vi "Fibonacci LFSRs -pseudo random.vi"() -> (3 "rand number":u16)   [LabVIEW 2021]
doc: "genarate pasodo random number.\nhttps://en.wikipedia.org/wiki/Linear-feedback_shift_register"
panel:
  # "tested, its has a flat histogram!"
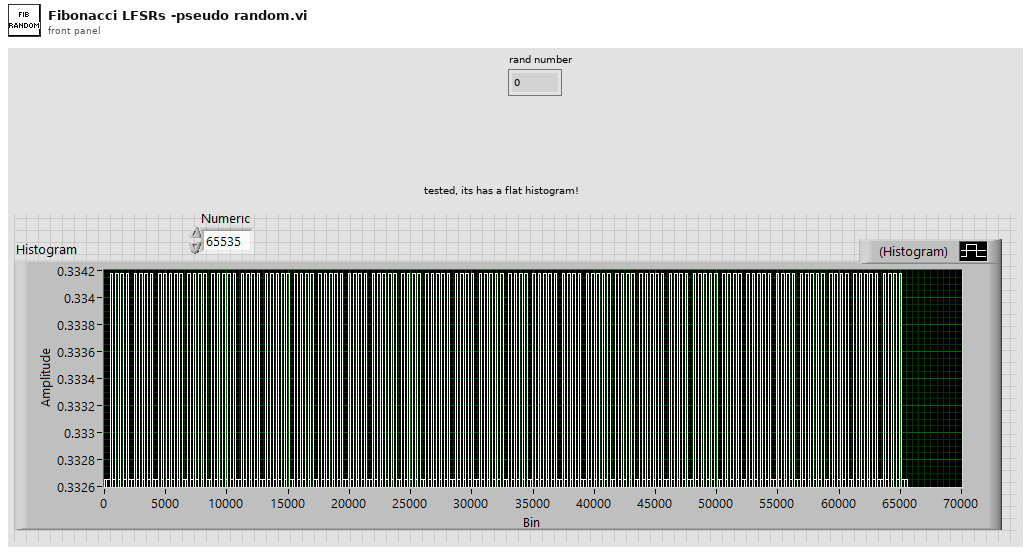
[diagram p1: front panel]
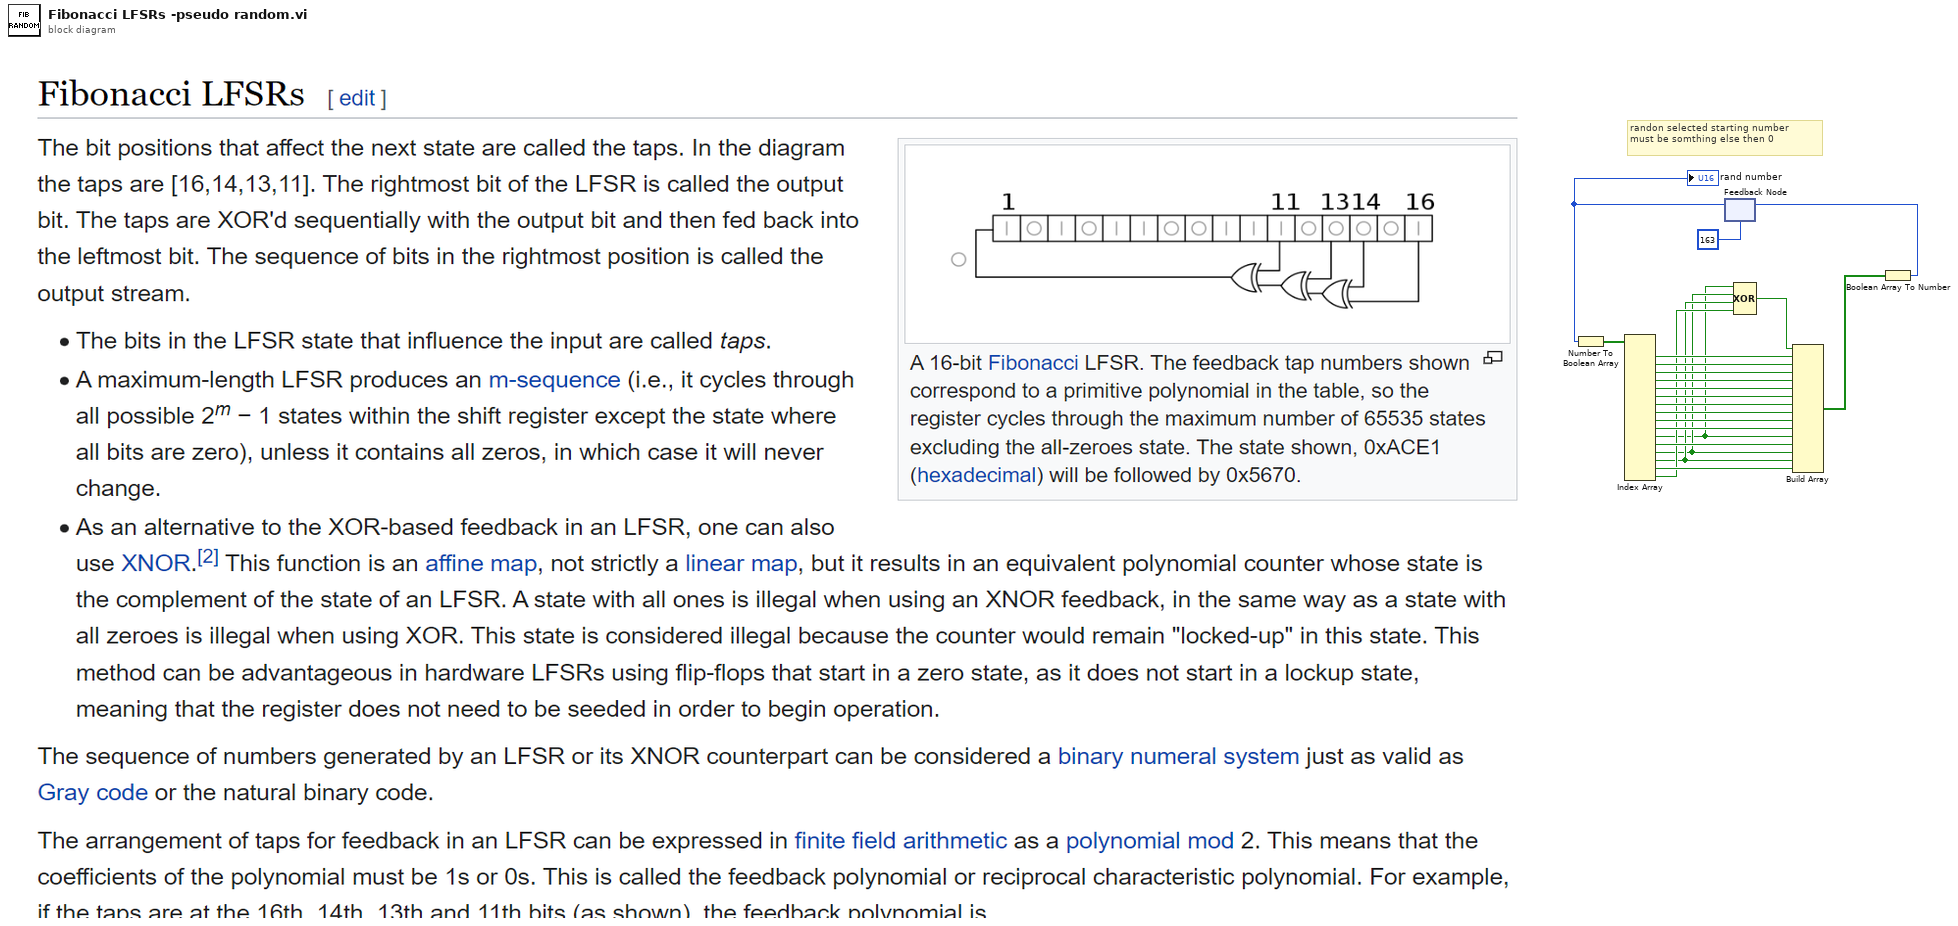
[diagram p0: block diagram]
diagram:
  # "randon selected starting number\nmust be somthing else then 0"
  n1 = feedback #1(u16 163) -> (w2:u16)
  "rand number" <- w2
  n2 = Number To Boolean Array(number=w2) -> (Boolean array=w22:bool[])
  n3 = Index Array(array=w22) -> (element #1=w20:bool, element #2=w19:bool, element #3=w18:bool, element #4=w17:bool, element #5=w16:bool, element #6=w15:bool, element #7=w14:bool, element #8=w13:bool, element #9=w12:bool, element #10=w11:bool, element #11=w5:bool, element #12=w10:bool, element #13=w6:bool, element #14=w7:bool, element #15=w9:bool, element #16=w8:bool)  [unwired: 16 in]
  n4 = Compound Arithmetic op=XOR(w5, w6, w7, w8) -> (w21:bool)
  n5 = Build Array(w21, w20, w19, w18, w17, w16, w15, w14, w13, w12, w11, w5, w10, w6, w7, w9) -> (w4:bool[])
  n6 = Boolean Array To Number(Boolean array=w4) -> (number=w3:u16)
  n7 = feedback-in #1(w3) -> ()
